vi "Boolean to Yes-No.vi"(1 "Bool":bool) -> (0 "Yes/No":string)   [LabVIEW 2011]
doc: "Returns true if string is empty.\n\n\nVersion 1.0 - 02/13/2013\n\nPhaeron, Inc.\nwww.phaeron.com\ninfo@phaeron.com"
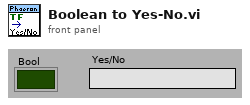
[diagram p1: front panel]
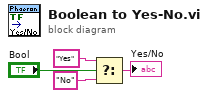
[diagram p0: block diagram]
diagram:
  n1 = Select(t="Yes", s="Bool", f="No") -> (s? t:f=→"Yes/No":string)
